vi "ziExample-HF2-PLL.vi"() -> ()   [LabVIEW 2009]
doc: "Control a Zurich instrument device via the LabOne Labview API. \nRequirements: Zurich Instruments HF2.\nThis example implements a simple PLL in LabVIEW.\n\n© Zurich Instruments AG, www.zhinst.com"
uses:
  <instrlib>/Zurich Instruments LabOne/Public/Utility/ziTicksToS_single.vi
  <instrlib>/Zurich Instruments LabOne/Zurich Instruments LabOne.lvlib
panel:
  out "Error Out":errorcluster
  out "output cluster":cluster{dbl[], dbl[]}
  out "Selected Device":string
  in  "Address":string="DEV"
  in  "DefaultSettings":bool
  in  "RefPhase":dbl=36.0 caption="Ref Phase (deg)"
  out "Error":dbl=0.0011898289611309565 format="%+8.5f°"
  out "Frequency":ext=1839836.4116389132 format="%_9pHz"
  out "Rate":dbl=94.24546185775438 format="%5.0pHz"
  in  "Gain":dbl(slide)=1.0 scale=0.1..1000.0 scale format="%#_6p"
  out "Phase":dbl=89.99881017103887 format="%+9.4g°"
  in  "CenterFreq":dbl=1838000.0 caption="Center Freq" format="%_6pHz"
  in  "SendFreq":bool
  out "Amplitude":dbl(graph)=1.0771498465688651
  out "Frequency":dbl(graph)
  in  "EnablePLL":bool=TRUE caption="Enable PLL"
  out "Timeconstant":dbl format="%#_3ps"
  out "Y":dbl=1.0771498463366156 format="%+_6pVrms"
  out "Amp":dbl=1.0771498465688651 format="%_6pVrms"
  out "X":dbl=2.2368173693618797e-05 format="%+_6pVrms"
  in  "Filter Order":u16=4
  in  "stop":bool=TRUE
  in  "Bandwidth":dbl=100.0
  # "Notes:\nCRYSTAL, HC-49/U, 1.8432MHZ; Frequenz, A\nIf signal very unstable: change gain (value of 1000 shows good stability), \nor check if you have the right peak (use set frequency and use the sweeper to find the right peak)\n\nThis PLL implmentation is very slow (more than 1000 times slower) compared to the PLL option that is \navailable for Zurich Instruments Lock-in Amplifiers. The PLL Option runs inside the instrument itself."
  # "Tested Instruments:\n- HF2LI"
  # "Filter Settings"
  # "PLL Settings"
  # "PLL Monitor"
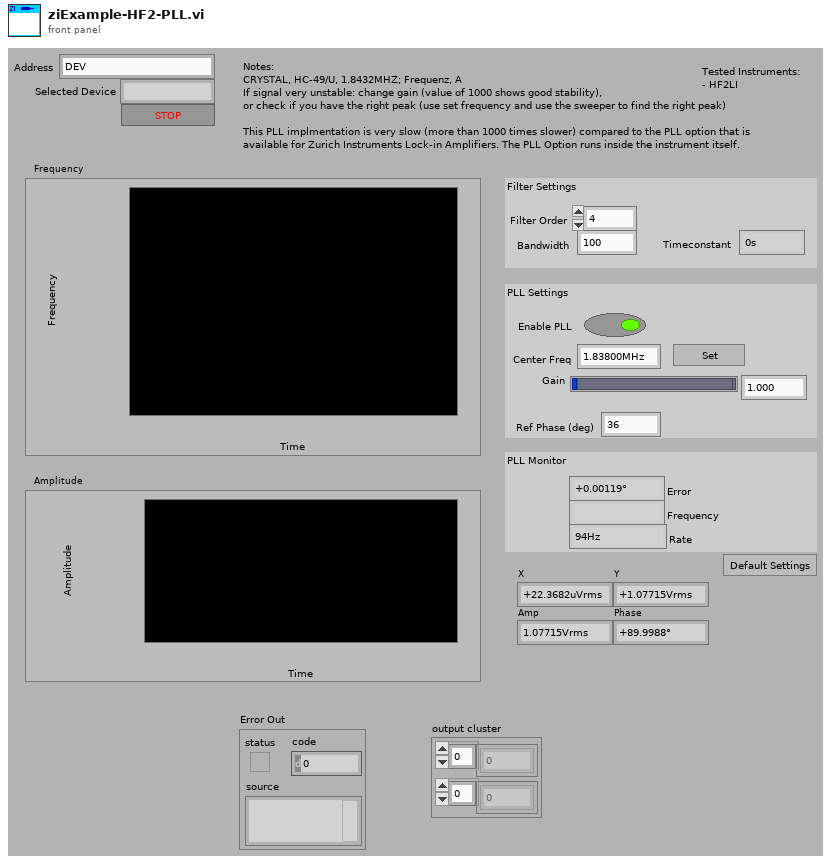
[diagram p1: front panel]
types:
  T1 = typedef "Zurich Instruments LabOne.lvlib/ziTypeHandle.ctl" = cluster{"handleValid":bool, "Conn":u64, "Path Prefix":string, "Handle":u64, "Connected":bool, "Clockbase(s)":dbl}
  T2 = cluster{"Timestamps (ticks)":u64, "X (Vrms)":dbl, "Y (Vrms)":dbl, "Osc Phase (deg)":dbl, "Freq (Hz)":dbl, "DIO":u32, "AuxIn0 (V)":dbl, "AuxIn1 (V)":dbl}
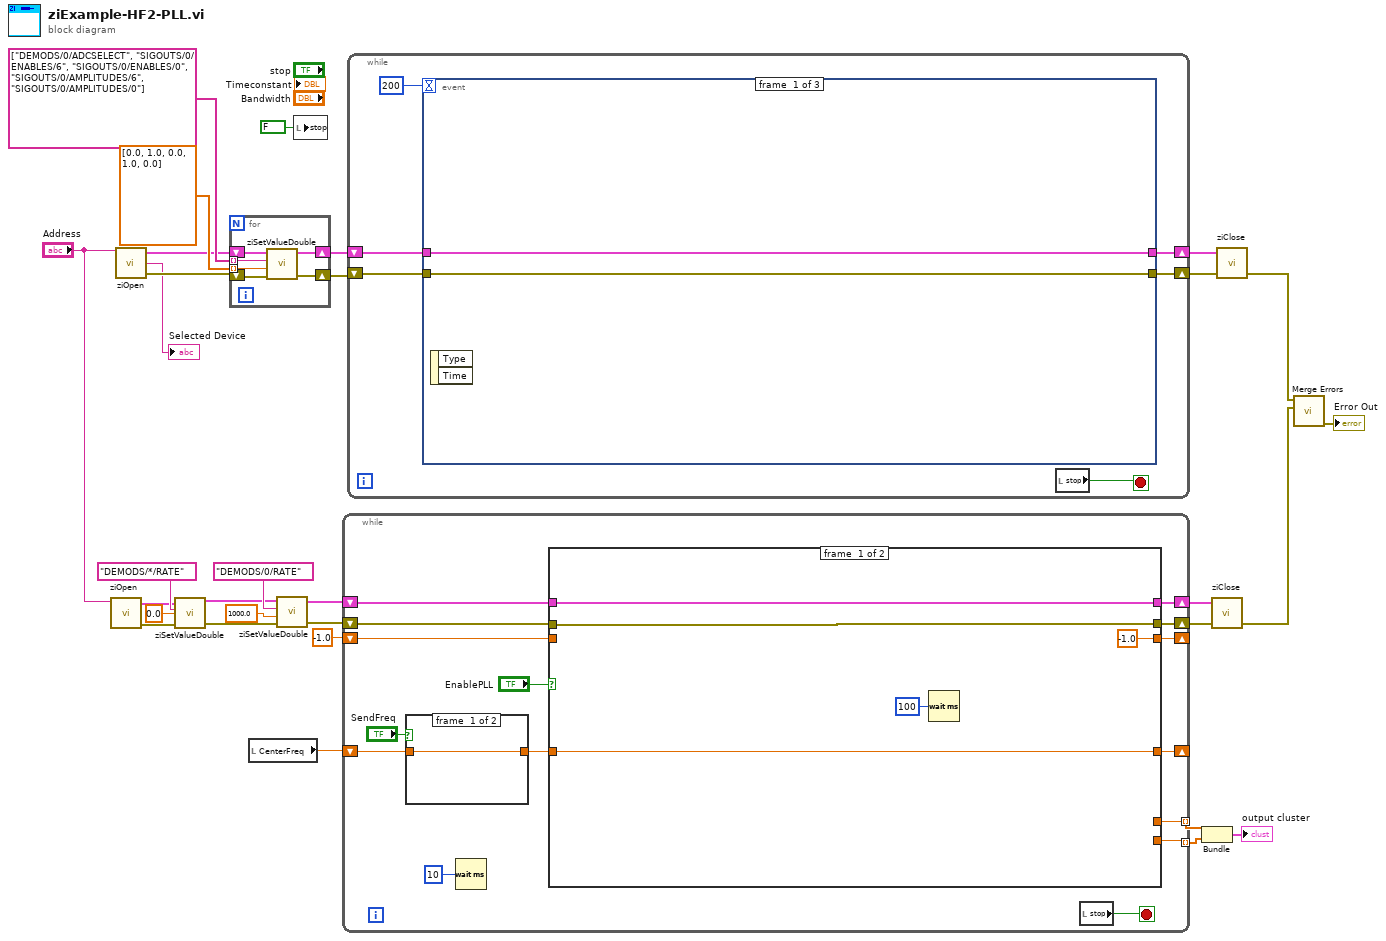
[diagram p0: block diagram]
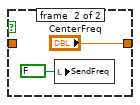
[diagram p2: hidden frame]
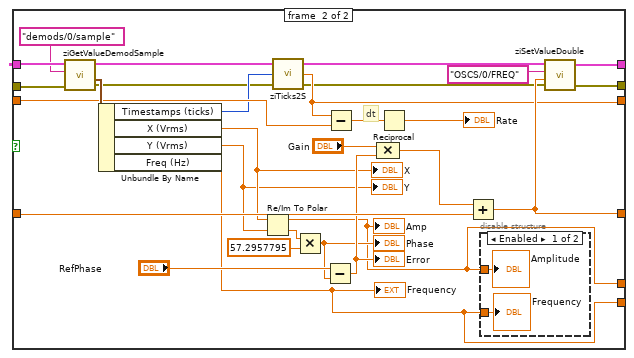
[diagram p3: hidden frame]
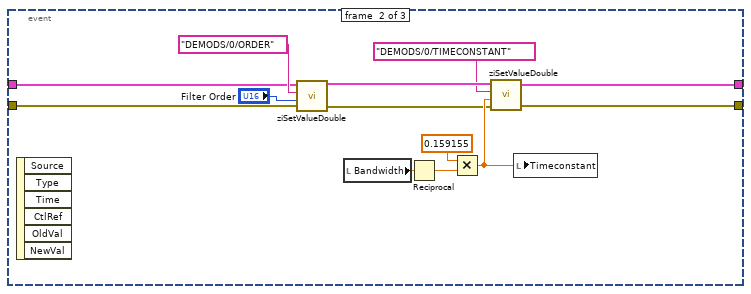
[diagram p5: hidden frame]
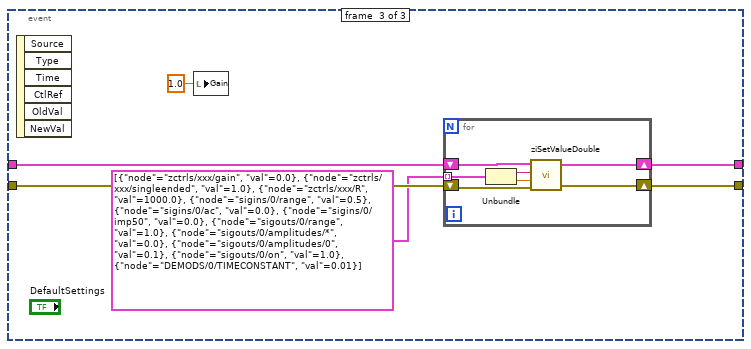
[diagram p6: hidden frame]
diagram:
  n1 = call <instrlib>:"ziOpen.vi"("Address"="Address") -> ("Error Out"=w19:errorcluster, "HandleOut"=w18:T1)  [unwired: 1 in, 3 out]
  n2 = call <instrlib>:"ziOpen.vi"("Address"="Address") -> ("Error Out"=w12:errorcluster, "Selected Device"=→"Selected Device":string, "HandleOut"=w11:T1)  [unwired: 1 in, 2 out]
  n3 = call <instrlib>:"ziSetValueDouble.vi"("Error In"=w19, "Value"=0.0, "Path"="DEMODS/*/RATE" ("Path (\"/\")"), "Handle In"=w18) -> ("Error Out"=w24:errorcluster, "Handle Out"=w23:T1)  [unwired: 1 out]
  n4 = for {
    tunnel: string[] ["DEMODS/0/ADCSELECT", "SIGOUTS/0/ENABLES/6", "SIGOUTS/0/ENABLES/0", "SIGOUTS/0/AMPLITUDES/6", "SIGOUTS/0/AMPLITUDES/0"] -> [w34] mode=indexing
    tunnel: dbl[] [0.0, 1.0, 0.0, 1.0, 0.0] -> [w33] mode=indexing
    shift-right: [w36] -> w10
    shift-left: w11 -> [w37]
    shift-right: [w35] -> w9
    shift-left: w12 -> [w32]
    n5 = call <instrlib>:"ziSetValueDouble.vi"("Error In"=w32, "Value"=w33, "Path"=w34, "Handle In"=w37) -> ("Error Out"=w35:errorcluster, "Handle Out"=w36:T1)  [unwired: 1 out]
  }
  n6 = local read "CenterFreq"() -> (w20:dbl)
  n7 = call <instrlib>:"ziSetValueDouble.vi"("Error In"=w24, "Value"=1000.0, "Path"="DEMODS/0/RATE" ("Path (\"/\")"), "Handle In"=w23) -> ("Error Out"=w17:errorcluster, "Handle Out"=w16:T1)  [unwired: 1 out]
  n8 = local write "stop"(FALSE ("stop")) -> ()
  n9 = while {
    shift-right: [w49] -> _
    shift-left: w20 -> [w47]
    shift-right: [w52] -> w26
    shift-left: w16 -> [w44]
    shift-right: [w51] -> w25
    shift-left: w17 -> [w45]
    shift-right: [w41] -> _
    shift-left: -1.0 ("Timestamps (s)") -> [w42]
    tunnel: [w39] -> w5 mode=indexing
    tunnel: [w38] -> w6 mode=indexing
    stop <- w50 stop-if-true
    n10 = case shown="True" "SendFreq" {
      tunnel: w47 -> [w53 _]
      tunnel: [w53 "CenterFreq"] -> w46
      frame #0 {
      }
      frame #1 {
        n11 = local write "SendFreq"(FALSE ("Set Frequency (PLL off)")) -> ()
      }
    }
    n12 = Wait (ms)(milliseconds to wait=u32 10) -> ()  [unwired: 1 out]
    n13 = case shown="True" "EnablePLL" {
      tunnel: w44 -> [w60 w81]
      tunnel: w45 -> [w59 w80]
      tunnel: [w60 w86] -> w52
      tunnel: [w59 w87] -> w51
      tunnel: w46 -> [w58 w89]
      tunnel: [w58 w85] -> w49
      tunnel: w42 -> [_ w74]
      tunnel: [-1.0 ("Timestamps (s)") w67] -> w41
      tunnel: [_ w62] -> w38
      tunnel: [_ w61] -> w39
      frame #0 {
        n14 = Wait (ms)(milliseconds to wait=u32 100) -> ()  [unwired: 1 out]
      }
      frame #1 {
        # "dt"
        n15 = call <instrlib>:"ziGetValueDemodSample.vi"("error in"=w80, "Path"="demods/0/sample" ("Path ()"), "Handle In"=w81) -> ("error out"=w64:errorcluster, "Demod Sample Out"=w77:T2, "Handle Out"=w66:T1)  [unwired: 1 in, 1 out]
        n16 = Unbundle By Name(w77) -> ("Timestamps (ticks)"=w68:u64, "X (Vrms)"=w76:dbl, "Y (Vrms)"=w75:dbl, "Freq (Hz)"=w61:dbl)
        "X" <- w76
        "Y" <- w75
        "Frequency" <- w61
        n17 = Re/Im To Polar(2:w75, 3:w76) -> (0:w84:dbl, 1:w62:dbl)
        "Amp" <- w62
        n18 = call-poly <instrlib>:"ziTicks2S.vi"("Error In"=w64, "Timestamp(ticks)"=w68, "Handle In"=w66) -> ("Error Out"=w63:errorcluster, "Timestamp(s)"=w67:dbl, "Handle Out"=w65:T1)
        n19 = Multiply(x=w84, y=57.2957795) -> (x*y=w70:dbl)
        "Phase" <- w70
        n20 = Subtract(x="RefPhase", y=w70) -> (x-y=w78:dbl)
        "Error" <- w78
        n21 = Subtract(x=w67, y=w74) -> (x-y=w69:dbl)
        n22 = Compound Arithmetic op=MULTIPLY("Gain", w78) -> (w71:dbl)
        n23 = Reciprocal(x=w69) -> (1/x=→"Rate":dbl)
        n24 = Add(x=w71, y=w89) -> (x+y=w85:dbl)
        n25 = disable-structure shown="Enabled" {
          disable-tunnel: w61 -> [w91 _]
          disable-tunnel: w62 -> [w90 _]
          frame #0 {
            "Frequency" <- w91
            "Amplitude" <- w90
          }
          frame #1 {
          }
        }
        n26 = call <instrlib>:"ziSetValueDouble.vi"("Error In"=w63, "Value"=w85, "Path"="OSCS/0/FREQ" ("name (unnamed)"), "Handle In"=w65) -> ("Error Out"=w87:errorcluster, "Handle Out"=w86:T1)  [unwired: 1 out]
      }
    }
    n27 = local read "stop"() -> (w50:bool)
  }
  n28 = while {
    shift-right: [w93] -> w28
    shift-left: w10 -> [w95]
    shift-right: [w92] -> w27
    shift-left: w9 -> [w94]
    stop <- w96 stop-if-true
    n29 = event shown="[1] \"Bandwidth\", \"Filter Order\": Value Change" {
      selector: _ -> [_ _ _]
      dyn-events: _ -> [_ _ _]
      timeout: 200 -> [_ _ _]
      tunnel: w95 -> [w99 w101 w116]
      tunnel: w94 -> [w98 w100 w115]
      tunnel: [w99 w103 w118] -> w93
      tunnel: [w98 w102 w117] -> w92
      event #0 {
        n30 = event-data() -> ()  [unwired: 3 out]
      }
      event #1 {
        n31 = event-data() -> ()  [unwired: 7 out]
        n32 = call <instrlib>:"ziSetValueDouble.vi"("Error In"=w100, "Value"="Filter Order", "Path"="DEMODS/0/ORDER" ("name (unnamed)"), "Handle In"=w101) -> ("Error Out"=w109:errorcluster, "Handle Out"=w108:T1)  [unwired: 1 out]
        n33 = local read "Bandwidth"() -> (w107:dbl)
        n34 = Reciprocal(x=w107) -> (1/x=w106:dbl)
        n35 = Multiply(x=0.159155 ("y"), y=w106) -> (x*y=w112:dbl)
        n36 = call <instrlib>:"ziSetValueDouble.vi"("Error In"=w109, "Value"=w112, "Path"="DEMODS/0/TIMECONSTANT" ("name (unnamed)"), "Handle In"=w108) -> ("Error Out"=w102:errorcluster, "Handle Out"=w103:T1)  [unwired: 1 out]
        n37 = local write "Timeconstant"(w112) -> ()
      }
      event #2 {
        n38 = event-data() -> ()  [unwired: 7 out]
        n39 = local write "Gain"(1.0 ("Gain")) -> ()
        n40 = for {
          tunnel: cluster{"node":string, "val":dbl}[] [{"node"="zctrls/xxx/gain", "val"=0.0}, {"node"="zctrls/xxx/singleended", "val"=1.0}, {"node"="zctrls/xxx/R", "val"=1000.0}, {"node"="sigins/0/range", "val"=0.5}, {"node"="sigins/0/ac", "val"=0.0}, {"node"="sigins/0/imp50", "val"=0.0}, {"node"="sigouts/0/range", "val"=1.0}, {"node"="sigouts/0/amplitudes/*", "val"=0.0}, {"node"="sigouts/0/amplitudes/0", "val"=0.1}, {"node"="sigouts/0/on", "val"=1.0}, {"node"="DEMODS/0/TIMECONSTANT", "val"=0.01}] -> [w121] mode=indexing
          shift-right: [w124] -> w118
          shift-left: w116 -> [w125]
          shift-right: [w123] -> w117
          shift-left: w115 -> [w122]
          n41 = Unbundle(w121) -> ("node"=w120:string, "val"=w119:dbl)
          n42 = call <instrlib>:"ziSetValueDouble.vi"("Error In"=w122, "Value"=w119, "Path"=w120, "Handle In"=w125) -> ("Error Out"=w123:errorcluster, "Handle Out"=w124:T1)  [unwired: 1 out]
        }
      }
    }
    n43 = local read "stop"() -> (w96:bool)
  }
  n44 = Bundle(w6, w5) -> (→"output cluster":cluster{dbl[], dbl[]})  [unwired: 1 in]
  n45 = call <instrlib>:"ziClose.vi"("Error In"=w25, "Handle In"=w26) -> ("Error Out"=w2:errorcluster)  [unwired: 3 out]
  n46 = call <instrlib>:"ziClose.vi"("Error In"=w27, "Handle In"=w28) -> ("Error Out"=w3:errorcluster)  [unwired: 3 out]
  n47 = call <vilib>:"Merge Errors.vi"("error in 2 (no error)"=w2, "error in 1 (no error)"=w3) -> ("error out"=→"Error Out":errorcluster)  [unwired: 5 in]
